vi "ObjectDefaults_testingOnly.vi"() -> ()   [LabVIEW 2012]
uses:
  ColumnVIs/Column/Column.lvclass
  ColumnVIs/DigitalCol/DigitalCol.lvclass
  ColumnVIs/SingleValCol/SingleValCol.lvclass
  ColumnVIs/TriggerCol/TriggerCol.lvclass
  Globals/DisabledColorGlobal.vi
  ColumnVIs/GroupCol/GroupCol.lvclass
  ColumnVIs/ModeCOl/ModeCol.lvclass
panel:
  in  "Trig isVariable?":bool
  in  "Mode isVariable?":bool
  out "GroupCol":refnum<class "GroupCol.lvclass">
  in  "Group Label":string="Group"
  in  "Group Text":u32[](array[colorbox])=[16448250, 0, 0]
  in  "Group Bkgd":u32[](array[colorbox])=[4194432, 10832639, 12880127]
  in  "Group Width":i32=40
  in  "Col Label":string
  out "Mode Col":refnum<class "ModeCol.lvclass">
  in  "Mode Disableable?":bool
  in  "Mode Label":string="Mode"
  in  "Mode Text":u32[](array[colorbox])=[0]
  in  "Mode Bkgd":u32[](array[colorbox])=[15326390]
  in  "Mode Width":i32=40
  out "Disableable Col":refnum<class "Column.lvclass">
  out "Non-disableable Col":refnum<class "Column.lvclass">
  out "Trig Col":refnum<class "TriggerCol.lvclass">
  in  "Trig Disableable?":bool
  in  "Trig Label":string
  in  "Trig Width":i32=10
  out "SingleVal Col":refnum<class "SingleValCol.lvclass">
  in  "Single Disableable?":bool
  in  "Single Label":string="nova2/3"
  in  "Single Text":u32[](array[colorbox])=[0]
  in  "Single Bkgd":u32[](array[colorbox])=[16448250]
  in  "Single Width":i32=60
  in  "Dig Label":string
  in  "Dig Text":u32[](array[colorbox])=[16448250, 0, 0]
  in  "Dig Bkgd":u32[](array[colorbox])=[1985280, 6618880, 14090026]
  out "Disableable Dig Col":refnum<class "DigitalCol.lvclass">
  out "Non-disableable Dig Col":refnum<class "DigitalCol.lvclass">
  in  "Digital Width":i32=18
  # "Column.lvclass defaults can also \nbe set in Column.ctl (since that's\nwhere the private data lives)"
  # "These default objects are ONLY intended for testing.\nWhen actually used, these column settings should be make when configuring Device.\n\nTo make new defaults, adjust settings and run the VI. Then right-click on the object you\nwant to use, Data Operations -> Make Current Values Default. You can then drag into\na TESTING vi.\n\nI prefer not to do this normally as the only way to determine the values (or type if\nupcast!) is to use a probe..."
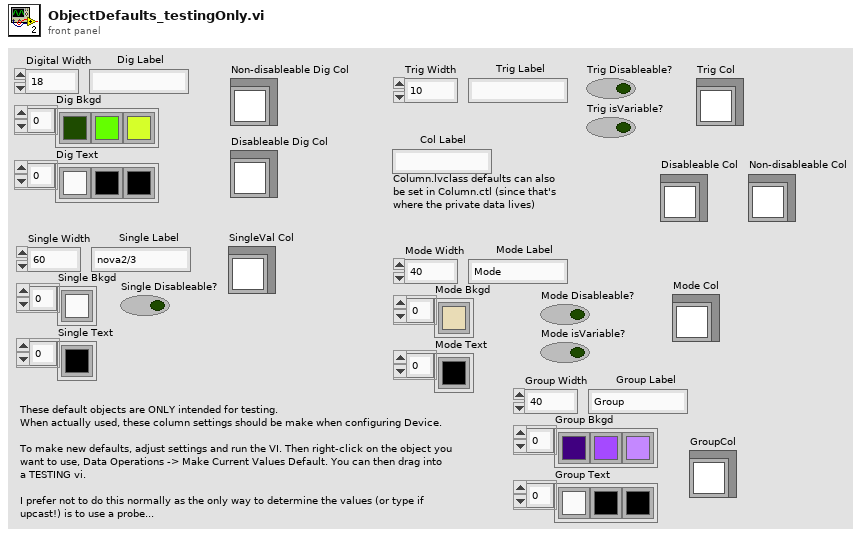
[diagram p1: front panel]
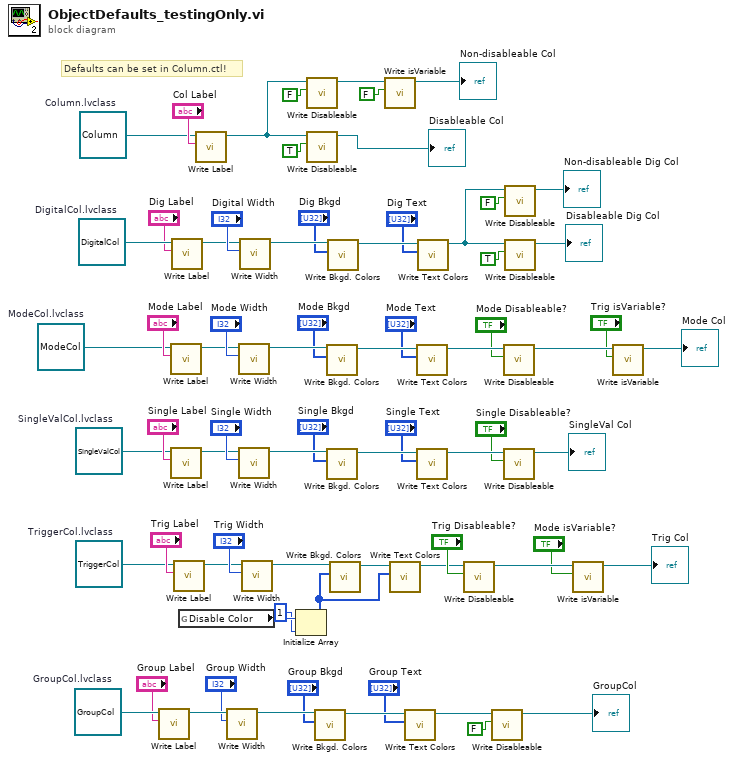
[diagram p0: block diagram]
diagram:
  w1 = refnum<class "ModeCol.lvclass"> refnum  # ModeCol.lvclass
  w16 = refnum<class "GroupCol.lvclass"> refnum  # GroupCol.lvclass
  w42 = refnum<class "TriggerCol.lvclass"> refnum  # TriggerCol.lvclass
  w49 = refnum<class "SingleValCol.lvclass"> refnum  # SingleValCol.lvclass
  w23 = refnum<class "Column.lvclass"> refnum  # Column.lvclass
  w65 = refnum<class "DigitalCol.lvclass"> refnum  # DigitalCol.lvclass
  # "Defaults can be set in Column.ctl!"
  n1 = call "Write Label.vi"("Label"="Group Label", "Column in"=w16) -> ("Column out"=w18:refnum<class "GroupCol.lvclass">)  [unwired: 8 in, 1 out]
  n2 = call "Write Label.vi"("Label"="Mode Label", "Column in"=w1) -> ("Column out"=w30:refnum<class "ModeCol.lvclass">)  [unwired: 8 in, 1 out]
  n3 = call "Write Label.vi"("Label"="Single Label", "Column in"=w49) -> ("Column out"=w52:refnum<class "SingleValCol.lvclass">)  [unwired: 8 in, 1 out]
  n4 = call "Write Label.vi"("Label"="Dig Label", "Column in"=w65) -> ("Column out"=w64:refnum<class "DigitalCol.lvclass">)  [unwired: 8 in, 1 out]
  n5 = call "Write Label.vi"("Label"="Trig Label", "Column in"=w42) -> ("Column out"=w45:refnum<class "TriggerCol.lvclass">)  [unwired: 8 in, 1 out]
  n6 = global read "DisabledColorGlobal.vi" "Disable Color"() -> (w41:u32)
  n7 = call "Write Label.vi"("Label"="Col Label", "Column in"=w23) -> ("Column out"=w22:refnum<class "Column.lvclass">)  [unwired: 8 in, 1 out]
  n8 = call "Write Width.vi"("Width"="Group Width", "Column in"=w18) -> ("Column out"=w21:refnum<class "GroupCol.lvclass">)  [unwired: 8 in, 1 out]
  n9 = call "Write Width.vi"("Width"="Mode Width", "Column in"=w30) -> ("Column out"=w35:refnum<class "ModeCol.lvclass">)  [unwired: 8 in, 1 out]
  n10 = call "Write Width.vi"("Width"="Single Width", "Column in"=w52) -> ("Column out"=w57:refnum<class "SingleValCol.lvclass">)  [unwired: 8 in, 1 out]
  n11 = call "Write Width.vi"("Width"="Digital Width", "Column in"=w64) -> ("Column out"=w70:refnum<class "DigitalCol.lvclass">)  [unwired: 8 in, 1 out]
  n12 = call "Write Width.vi"("Width"="Trig Width", "Column in"=w45) -> ("Column out"=w46:refnum<class "TriggerCol.lvclass">)  [unwired: 8 in, 1 out]
  n13 = Initialize Array(w41, 1 ("dimension size")) -> (w25:u32[])
  n14 = call "Write Disableable.vi"("Disableable?"=FALSE, "Column in"=w22) -> ("Column out"=w4:refnum<class "Column.lvclass">)  [unwired: 8 in, 1 out]
  n15 = call "Write Disableable.vi"("Disableable?"=TRUE, "Column in"=w22) -> ("Column out"=→"Disableable Col":refnum<class "Column.lvclass">)  [unwired: 8 in, 1 out]
  n16 = call "Write Bkgd. Colors.vi"("Bkgd. Colors"="Group Bkgd", "Column in"=w21) -> ("Column out"=w20:refnum<class "GroupCol.lvclass">)  [unwired: 8 in, 1 out]
  n17 = call "Write Bkgd. Colors.vi"("Bkgd. Colors"="Mode Bkgd", "Column in"=w35) -> ("Column out"=w34:refnum<class "ModeCol.lvclass">)  [unwired: 8 in, 1 out]
  n18 = call "Write Bkgd. Colors.vi"("Bkgd. Colors"="Single Bkgd", "Column in"=w57) -> ("Column out"=w56:refnum<class "SingleValCol.lvclass">)  [unwired: 8 in, 1 out]
  n19 = call "Write Bkgd. Colors.vi"("Bkgd. Colors"="Dig Bkgd", "Column in"=w70) -> ("Column out"=w69:refnum<class "DigitalCol.lvclass">)  [unwired: 8 in, 1 out]
  n20 = call "Write Bkgd. Colors.vi"("Bkgd. Colors"=w25, "Column in"=w46) -> ("Column out"=w27:refnum<class "TriggerCol.lvclass">)  [unwired: 8 in, 1 out]
  n21 = call "Write isVariable.vi"("isVariable?"=FALSE, "Column in"=w4) -> ("Column out"=→"Non-disableable Col":refnum<class "Column.lvclass">)  [unwired: 8 in, 1 out]
  n22 = call "Write Text Colors.vi"("Text Colors"=w25, "Column in"=w27) -> ("Column out"=w26:refnum<class "TriggerCol.lvclass">)  [unwired: 8 in, 1 out]
  n23 = call "Write Text Colors.vi"("Text Colors"="Group Text", "Column in"=w20) -> ("Column out"=w19:refnum<class "GroupCol.lvclass">)  [unwired: 8 in, 1 out]
  n24 = call "Write Text Colors.vi"("Text Colors"="Mode Text", "Column in"=w34) -> ("Column out"=w31:refnum<class "ModeCol.lvclass">)  [unwired: 8 in, 1 out]
  n25 = call "Write Text Colors.vi"("Text Colors"="Single Text", "Column in"=w56) -> ("Column out"=w53:refnum<class "SingleValCol.lvclass">)  [unwired: 8 in, 1 out]
  n26 = call "Write Text Colors.vi"("Text Colors"="Dig Text", "Column in"=w69) -> ("Column out"=w66:refnum<class "DigitalCol.lvclass">)  [unwired: 8 in, 1 out]
  n27 = call "Write Disableable.vi"("Disableable?"="Trig Disableable?", "Column in"=w26) -> ("Column out"=w10:refnum<class "TriggerCol.lvclass">)  [unwired: 8 in, 1 out]
  n28 = call "Write Disableable.vi"("Disableable?"=FALSE, "Column in"=w19) -> ("Column out"=→"GroupCol":refnum<class "GroupCol.lvclass">)  [unwired: 8 in, 1 out]
  n29 = call "Write Disableable.vi"("Disableable?"="Mode Disableable?", "Column in"=w31) -> ("Column out"=w7:refnum<class "ModeCol.lvclass">)  [unwired: 8 in, 1 out]
  n30 = call "Write Disableable.vi"("Disableable?"="Single Disableable?", "Column in"=w53) -> ("Column out"=→"SingleVal Col":refnum<class "SingleValCol.lvclass">)  [unwired: 8 in, 1 out]
  n31 = call "Write Disableable.vi"("Disableable?"=FALSE, "Column in"=w66) -> ("Column out"=→"Non-disableable Dig Col":refnum<class "DigitalCol.lvclass">)  [unwired: 8 in, 1 out]
  n32 = call "Write Disableable.vi"("Disableable?"=TRUE, "Column in"=w66) -> ("Column out"=→"Disableable Dig Col":refnum<class "DigitalCol.lvclass">)  [unwired: 8 in, 1 out]
  n33 = call "Write isVariable.vi"("isVariable?"="Mode isVariable?", "Column in"=w10) -> ("Column out"=→"Trig Col":refnum<class "TriggerCol.lvclass">)  [unwired: 8 in, 1 out]
  n34 = call "Write isVariable.vi"("isVariable?"="Trig isVariable?", "Column in"=w7) -> ("Column out"=→"Mode Col":refnum<class "ModeCol.lvclass">)  [unwired: 8 in, 1 out]
